vi "Construct Network Session Handler.vi"(6 "Log Instance":refnum<class "LoggerReference.lvclass">, 8 "Log Alias":string, 9 "Max Number of Connections":i32, 10 "MessageProtocol":refnum<class "IMessagingProtocol.lvclass">, 11 "Connection Factory":refnum<class "IConnectionFactory.lvclass">) -> (0 "error out":errorcluster, 2 "Read Queue":refnum<queue>, 3 "Session Queue":refnum<class "Message Queue.lvclass">)   [LabVIEW 2017, in "Network Interface.lvlib" / "Network Session Handler.lvclass"]
uses:
  <vilib>/gpm_packages/@cs/Network-sink/Source/Network Interface/Network Session Handler/Network Session Handler.lvclass
  <vilib>/gpm_packages/@cs/Network-sink/Source/Network Interface/IConnectionFactory/IConnectionFactory.lvclass
  <vilib>/gpm_packages/@cs/Network-sink/Source/Network Interface/IMessagingProtocol/IMessagingProtocol.lvclass
  <vilib>/gpm_packages/@cs/Network-sink/Source/Network Interface/Message Queue/Message Queue.lvclass
  <vilib>/gpm_packages/@cs/event-logger/Source/Composed Log/LoggerReference/LoggerReference.lvclass
  <vilib>/gpm_packages/@cs/Network-sink/Source/Network Interface/Network Session Handler/Network Session Handler.lvclass/Network Session Handler.ctl
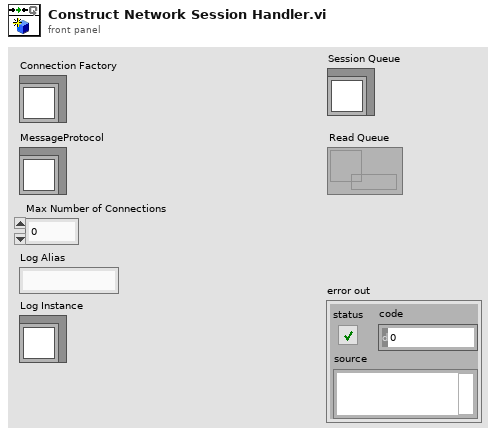
[diagram p1: front panel]
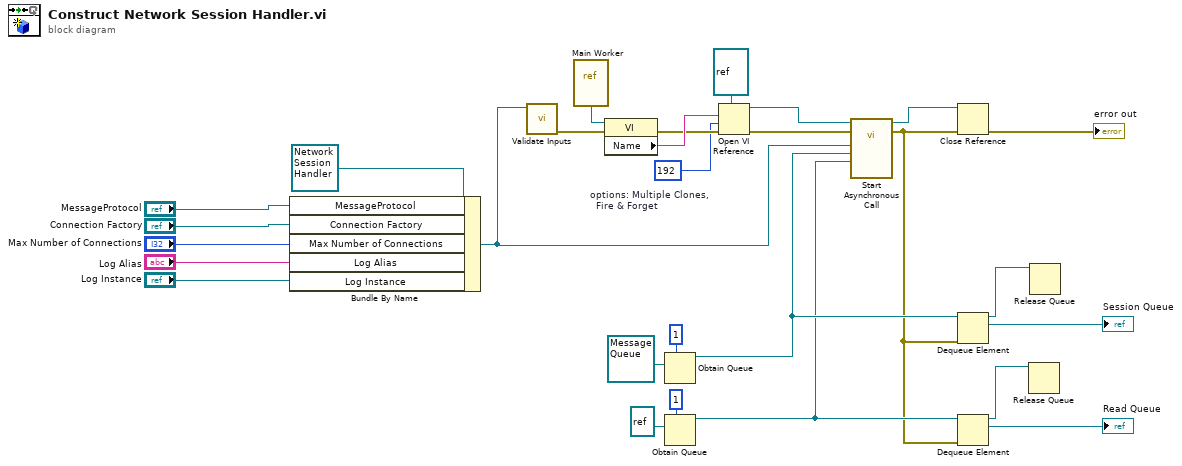
[diagram p0: block diagram]
diagram:
  w6 = 192  # options: Multiple Clones,   Fire & Forget
  n1 = Bundle By Name(cluster=refnum<class "Network Session Handler.lvclass"> refnum ("Connection Factory Session in"), "MessageProtocol"="MessageProtocol", "Connection Factory"="Connection Factory", "Max Number of Connections"="Max Number of Connections", "Log Alias"="Log Alias", "Log Instance"="Log Instance") -> (w2:refnum<class "Network Session Handler.lvclass">)
  n2 = call <vilib>:"Validate Inputs.vi"("Network Session Handler in"=w2) -> ("error out"=w1:errorcluster)  [unwired: 10 in]
  n3 = vi-ref <vilib>:"Main Worker.vi"() -> (w22:refnum<vi>)
  n4 = property class="VI"(reference=w22, error in=w1) -> (error out=w17:errorcluster, "Name"=w21:string)  [unwired: 1 out]
  n5 = Obtain Queue(max queue size (-1, unlimited)=1, element data type=refnum<class "Message Queue.lvclass"> refnum ("Controller Queue")) -> (queue out=w14:refnum<queue>)  [unwired: 3 in, 2 out]
  n6 = Obtain Queue(max queue size (-1, unlimited)=1, element data type=refnum<queue> refnum ("queue out")) -> (queue out=w13:refnum<queue>)  [unwired: 3 in, 2 out]
  n7 = Open VI Reference(type specifier VI Refnum (for type only)=refnum<vi> refnum, vi path=w21, options=w6, error in (no error)=w17) -> (vi reference=w19:refnum<vi>, error out=w18:errorcluster)  [unwired: 2 in]
  n8 = call-by-ref "Start Asynchronous Call"(reference=w19, error in=w18, "Read Queue Return"=w13, "Control Queue Return"=w14, "Connection Factory Session in"=w2) -> (reference out=w15:refnum<vi>, error out=w12:errorcluster)  [unwired: 9 in]
  n9 = Close Reference(reference=w15, error in (no error)=w12) -> (error out=→"error out":errorcluster)
  n10 = Dequeue Element(queue=w14, error in (no error)=w12) -> (queue out=w10:refnum<queue>, element=→"Session Queue":refnum<class "Message Queue.lvclass">)  [unwired: 1 in, 2 out]
  n11 = Dequeue Element(queue=w13, error in (no error)=w12) -> (queue out=w9:refnum<queue>, element=→"Read Queue":refnum<queue>)  [unwired: 1 in, 2 out]
  n12 = Release Queue(queue=w9) -> ()  [unwired: 2 in, 3 out]
  n13 = Release Queue(queue=w10) -> ()  [unwired: 2 in, 3 out]
